vi "get channels from function.vi"(11 "processing function":T1) -> (3 "channels":refnum<class "TBM channel.lvclass">[](array[class]))   [LabVIEW 2013, in "Logic Sequencer configuration.lvclass"]
uses:
  Logic Sequencer configuration.lvclass
  processing channels.ctl
  <vilib>/NI/Tag Bus Module Framework/channel/TBM channel.lvclass
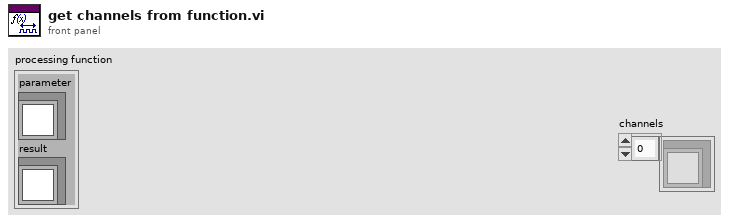
[diagram p1: front panel]
types:
  T1 = typedef "Logic Sequencer configuration.lvclass/processing channels.ctl" = cluster{"parameter":refnum<class "TBM channel.lvclass">, "result":refnum<class "TBM channel.lvclass">}
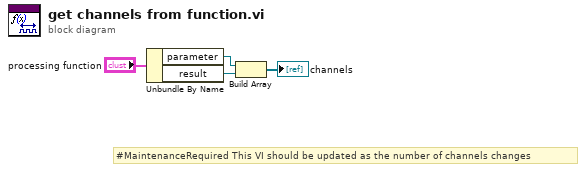
[diagram p0: block diagram]
diagram:
  # "#MaintenanceRequired This VI should be updated as the number of channels changes"
  n1 = Unbundle By Name("processing function") -> ("parameter"=w3:refnum<class "TBM channel.lvclass">, "result"=w2:refnum<class "TBM channel.lvclass">)
  n2 = Build Array(w3, w2) -> (→"channels":refnum<class "TBM channel.lvclass">[])
